vi "SolveMotor_Volts,Speed.vi"(8 "Reference Voltage (12)":dbl=12.0, 9 "Motor Characteristics":T2, 10 "Motor Speed":dbl, 11 "Motor Voltage":dbl) -> (3 "Motor Data":T1)   [LabVIEW 2014]
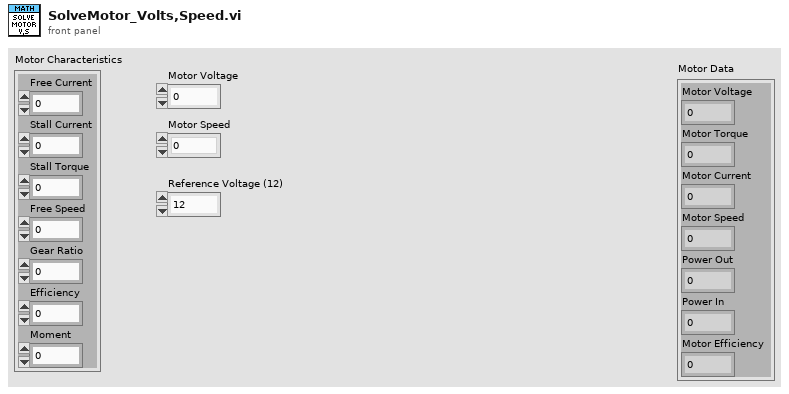
[diagram p1: front panel]
types:
  T1 = cluster{"Motor Voltage":dbl, "Motor Torque":dbl, "Motor Current":dbl, "Motor Speed":dbl, "Power Out":dbl, "Power In":dbl, "Motor Efficiency":dbl}
  T2 = cluster{"Free Current":dbl, "Stall Current":dbl, "Stall Torque":dbl, "Free Speed":dbl, "Gear Ratio":dbl, "Efficiency":dbl, "Moment":dbl}
  T3 = cluster{"[0]":dbl, "[1]":dbl, "[2]":dbl, "[3]":dbl, "[4]":dbl, "[5]":dbl, "[6]":dbl}
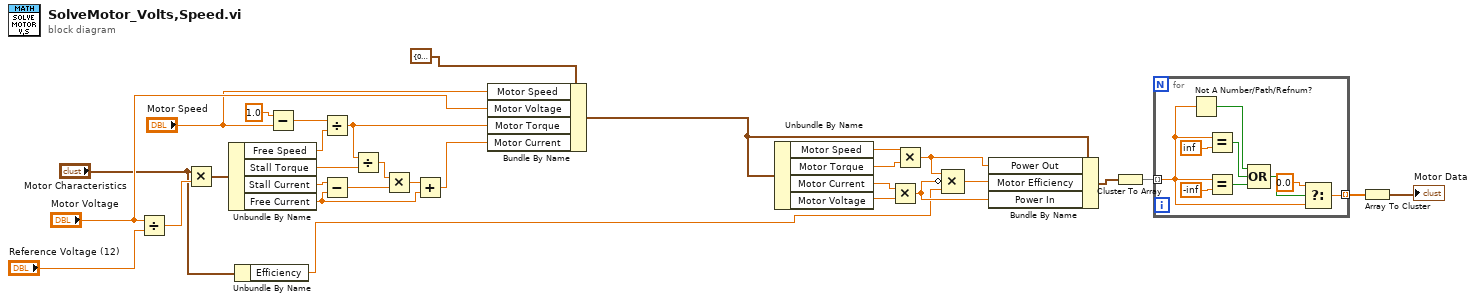
[diagram p0: block diagram]
diagram:
  n1 = Divide(x="Motor Voltage", y="Reference Voltage (12)") -> (x/y=w30:dbl)
  n2 = Multiply(x="Motor Characteristics", y=w30) -> (x*y=w29:T2)
  n3 = Unbundle By Name(w29) -> ("Free Speed"=w24:dbl, "Stall Torque"=w22:dbl, "Stall Current"=w21:dbl, "Free Current"=w17:dbl)
  n4 = Unbundle By Name("Motor Characteristics") -> ("Efficiency"=w5:dbl)
  n5 = Subtract(x=1.0, y="Motor Speed") -> (x-y=w25:dbl)
  n6 = Divide(x=w25, y=w24) -> (x/y=w23:dbl)
  n7 = Subtract(x=w21, y=w17) -> (x-y=w19:dbl)
  n8 = Divide(x=w23, y=w22) -> (x/y=w20:dbl)
  n9 = Multiply(x=w20, y=w19) -> (x*y=w18:dbl)
  n10 = Add(x=w18, y=w17) -> (x+y=w16:dbl)
  n11 = Bundle By Name(cluster=T1 {"Motor Voltage"=0.0, "Motor Torque"=0.0, "Motor Current"=0.0, "Motor Speed"=0.0, "Power Out"=0.0, "Power In"=0.0, "Motor Efficiency"=0.0} ("Motor Data 2"), "Motor Speed"="Motor Speed", "Motor Voltage"="Motor Voltage", "Motor Torque"=w23, "Motor Current"=w16) -> (w8:T1)
  n12 = Unbundle By Name(w8) -> ("Motor Speed"=w15:dbl, "Motor Torque"=w14:dbl, "Motor Current"=w12:dbl, "Motor Voltage"=w13:dbl)
  n13 = Multiply(x=w12, y=w13) -> (x*y=w9:dbl)
  n14 = Multiply(x=w15, y=w14) -> (x*y=w10:dbl)
  n15 = Compound Arithmetic op=MULTIPLY(w10, invert w9, w5) -> (w11:dbl)
  n16 = Bundle By Name(cluster=w8, "Power Out"=w10, "Motor Efficiency"=w11, "Power In"=w9) -> (w2:T1)
  n17 = Cluster To Array(cluster=w2) -> (array=w4:dbl[])
  n18 = for {
    tunnel: w4 -> [w37] mode=indexing
    tunnel: [w32] -> w3 mode=indexing
    n19 = Not A Number/Path/Refnum?(number/path/refnum=w37) -> (NaN/Path/Refnum?=w36:bool)
    n20 = Equal?(x=w37, y=inf) -> (x = y?=w34:bool)
    n21 = Equal?(x=w37, y=-inf) -> (x = y?=w35:bool)
    n22 = Compound Arithmetic op=OR(w36, w34, w35) -> (w33:bool)
    n23 = Select(t=0.0, s=w33, f=w37) -> (s? t:f=w32:dbl)
  }
  n24 = Array To Cluster(array=w3) -> (cluster=→"Motor Data":T3)
